vi "Open Connection+.vi"(6 "Options":i32, 8 "error in (no error)":errorcluster, 9 "Password":string, 10 "UserID":string, 11 "Connection String":string) -> (0 "error out":errorcluster, 2 "ADO Version":string, 3 "Connection":refnum<k7>)   [LabVIEW 2014, in "hse-db.lvlib" / "ADO-DB-Driver.lvlib"]
uses:
  ADO-DB-Driver.lvlib
panel:
  in  "?":refnum<k7>
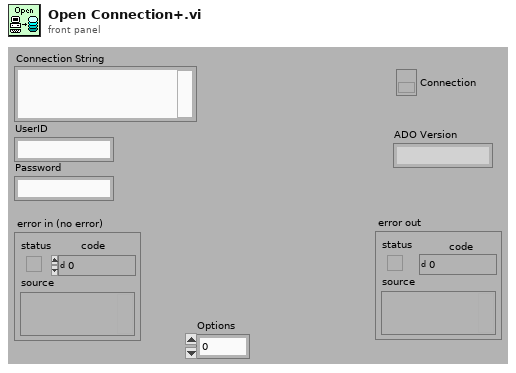
[diagram p1: front panel]
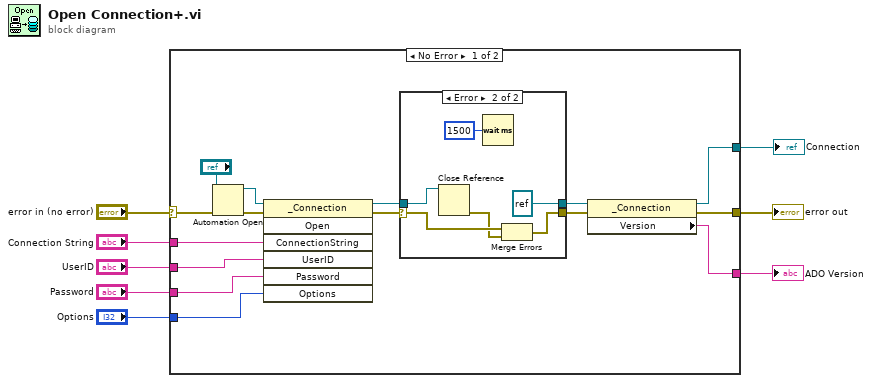
[diagram p0: block diagram]
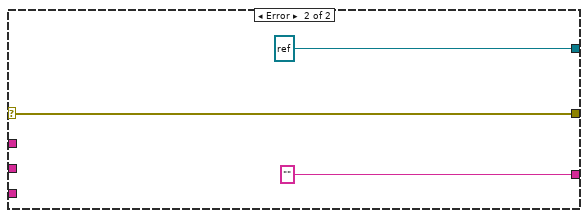
[diagram p3: hidden frame]
diagram:
  n1 = case shown="No Error" "error in (no error)" {
    selector: "error in (no error)" -> [w9 w34]
    tunnel: [w23 "" ("Version")] -> w8
    tunnel: "Connection String" -> [w20 _]
    tunnel: [w14 refnum<k7> refnum] -> w6
    tunnel: [w13 w34] -> w5
    tunnel: "UserID" -> [w12 _]
    tunnel: "Password" -> [w11 _]
    tunnel: "Options" -> [w10 _]
    frame No Error {
      n2 = Automation Open(error in (no error)=w9, Automation Refnum="?") -> (Automation Refnum=w17:refnum<k7>, error out=w18:errorcluster)  [unwired: 2 in]
      n3 = invoke class="_Connection" method="Open"(reference=w17, error in=w18, "ConnectionString"=w20, "UserID"=w12, "Password"=w11, "Options"=w10) -> (reference out=w15:refnum<k7>, error out=w16:errorcluster)  [unwired: 1 in, 5 out]
      n4 = case shown="Error" w16 {
        selector: w16 -> [w25 w28]
        tunnel: w15 -> [w24 w30]
        tunnel: [w25 w26] -> w22
        tunnel: [w24 refnum<k7> refnum] -> w21
        frame No Error {
        }
        frame Error {
          n5 = Close Reference(reference=w30) -> (error out=w27:errorcluster)  [unwired: 1 in]
          n6 = Wait (ms)(milliseconds to wait=u32 1500 ("Milliseconds to Delay")) -> ()  [unwired: 1 out]
          n7 = Merge Errors(w28, w27) -> (w26:errorcluster)
        }
      }
      n8 = property class="_Connection"(reference=w21, error in=w22) -> (reference out=w14:refnum<k7>, error out=w13:errorcluster, "Version"=w23:string)
    }
    frame Error {
    }
  }
  "error out" <- w5
  "ADO Version" <- w8
  "Connection" <- w6
